vi "SwitchGame.vi"(8 "error in (no error)":errorcluster, 11 "Engine in":refnum<class "Engine.lvclass">) -> (0 "error out":errorcluster, 3 "Engine out":refnum<class "Engine.lvclass">)   [LabVIEW 2019, in "RT_Game.lvlib" / "Engine.lvclass"]
uses:
  Engine.lvclass
  Game/Game.lvclass
  Engine.lvclass/Engine.ctl
  Game/Game.lvclass/Game.ctl
  Game/Read FlattenedNextClass.vi
  Game/Write StopMoveNotifier.vi
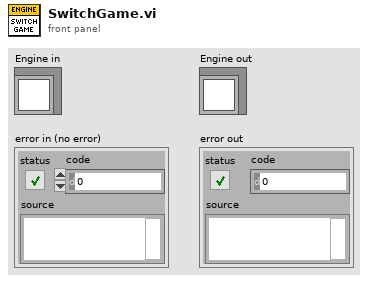
[diagram p1: front panel]
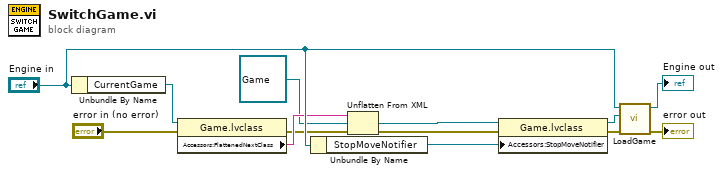
[diagram p0: block diagram]
diagram:
  n1 = Unbundle By Name("Engine in") -> ("CurrentGame"=w13:refnum<class "Game.lvclass">)
  n2 = property class="Game.lvclass"(reference=w13, error in="error in (no error)") -> (error out=w6:errorcluster, "Accessors:FlattenedNextClass"=w7:string)  [unwired: 1 out]
  n3 = Unbundle By Name("Engine in") -> ("StopMoveNotifier"=w11:refnum<notifier>)
  n4 = Unflatten From XML(xml string=w7, type=refnum<class "Game.lvclass"> refnum ("RT_Game.lvlib:Game.lvclass"), error in (no error)=w6) -> (value=w9:refnum<class "Game.lvclass">, error out=w3:errorcluster)
  n5 = property class="Game.lvclass"(reference=w9, error in=w3, "Accessors:StopMoveNotifier"=w11) -> (reference out=w10:refnum<class "Game.lvclass">, error out=w8:errorcluster)
  n6 = call "LoadGame.vi"("error in (no error)"=w8, "NewGame"=w10, "Engine in"="Engine in") -> ("error out"=→"error out":errorcluster, "Engine out"=→"Engine out":refnum<class "Engine.lvclass">)  [unwired: 7 in]
